vi "CheckArrowKeys.vi"(11 "Array":T1(array[ring])) -> (0 "Down":bool, 1 "Right":bool, 2 "Left":bool, 3 "Up":bool, 4 "Space":bool)   [LabVIEW 2019]
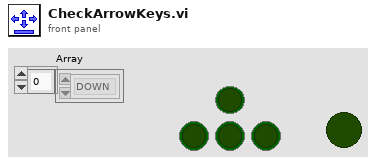
[diagram p1: front panel]
types:
  T1 = enum16{"0", "1", "2", "3", "4", "5", "6", "7", "8", "9", "A", "B", "C", "D", "E", "F", "G", "H", "I", "J", "K", "L", "M", "N", "O", "P", "Q", "R", "S", "T", "U", "V", "W", "X", "Y", "Z", "F1", "F2", "F3", "F4", "F5", "F6", "F7", "F8", "F9", "F10", "F11", "F12", "F13", "F14", "F15", "ADD", "BACK", "BACKSLASH", "CAPITAL", "COMMA", "DECIMAL", "DELETE", "DIVIDE", "DOWN", "END", "EQUALS", "ESCAPE", "GRAVE (`)", "HOME", "INSERT", "LBRACKET", "LCONTROL", "LEFT", "L ALT", "LSHIFT", "LWIN", "MINUS", "MULTIPLY", "NEXT", "NUMLOCK", "NUMPAD_0", "NUMPAD_1", "NUMPAD_2", "NUMPAD_3", "NUMPAD_4", "NUMPAD_5", "NUMPAD_6", "NUMPAD_7", "NUMPAD_8", "NUMPAD_9", "PAUSE", "PERIOD", "PRIOR (PG UP)", "RBRACKET", "RCONTROL", "RETURN", "RIGHT", "R ALT", "RSHIFT", "RWIN", "SCROLL", "SEMICOLON", "SLASH", "SPACE", "SUBTRACT", "TAB", "UP", "ENTER (num pad)", "' (quote)"}[]
  T2 = enum16{"0", "1", "2", "3", "4", "5", "6", "7", "8", "9", "A", "B", "C", "D", "E", "F", "G", "H", "I", "J", "K", "L", "M", "N", "O", "P", "Q", "R", "S", "T", "U", "V", "W", "X", "Y", "Z", "F1", "F2", "F3", "F4", "F5", "F6", "F7", "F8", "F9", "F10", "F11", "F12", "F13", "F14", "F15", "ADD", "BACK", "BACKSLASH", "CAPITAL", "COMMA", "DECIMAL", "DELETE", "DIVIDE", "DOWN", "END", "EQUALS", "ESCAPE", "GRAVE (`)", "HOME", "INSERT", "LBRACKET", "LCONTROL", "LEFT", "L ALT", "LSHIFT", "LWIN", "MINUS", "MULTIPLY", "NEXT", "NUMLOCK", "NUMPAD_0", "NUMPAD_1", "NUMPAD_2", "NUMPAD_3", "NUMPAD_4", "NUMPAD_5", "NUMPAD_6", "NUMPAD_7", "NUMPAD_8", "NUMPAD_9", "PAUSE", "PERIOD", "PRIOR (PG UP)", "RBRACKET", "RCONTROL", "RETURN", "RIGHT", "R ALT", "RSHIFT", "RWIN", "SCROLL", "SEMICOLON", "SLASH", "SPACE", "SUBTRACT", "TAB", "UP", "ENTER (num pad)", "' (quote)"}
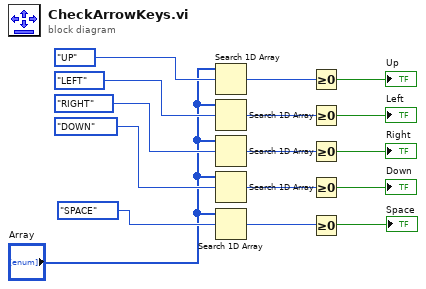
[diagram p0: block diagram]
diagram:
  n1 = Search 1D Array(1D array="Array", element=T2."UP" ("keys pressed[2]")) -> (index of element=w12:i32)  [unwired: 1 in]
  n2 = Search 1D Array(1D array="Array", element=T2."LEFT" ("keys pressed[0]")) -> (index of element=w11:i32)  [unwired: 1 in]
  n3 = Search 1D Array(1D array="Array", element=T2."RIGHT" ("keys pressed[1]")) -> (index of element=w10:i32)  [unwired: 1 in]
  n4 = Search 1D Array(1D array="Array", element=T2."DOWN" ("keys pressed[0]")) -> (index of element=w9:i32)  [unwired: 1 in]
  n5 = Search 1D Array(1D array="Array", element=T2."SPACE" ("keys pressed[0]")) -> (index of element=w3:i32)  [unwired: 1 in]
  n6 = Greater Or Equal To 0?(x=w12) -> (x >= 0?=→"Up":bool)
  n7 = Greater Or Equal To 0?(x=w11) -> (x >= 0?=→"Left":bool)
  n8 = Greater Or Equal To 0?(x=w10) -> (x >= 0?=→"Right":bool)
  n9 = Greater Or Equal To 0?(x=w9) -> (x >= 0?=→"Down":bool)
  n10 = Greater Or Equal To 0?(x=w3) -> (x >= 0?=→"Space":bool)
